vi "HydrophonePeaks.vi"() -> ()   [LabVIEW 2022 SP3]
uses:
  <vilib>/Analysis/NI_AALPro.lvlib
  <vilib>/Analysis/5stat.llb/RMS (DBL).vi
  <vilib>/Utility/file.llb/Write To Spreadsheet File (DBL).vi
panel:
  out "Waveform Graph 2":dbl[](graph)
  out "Waveform Graph":dbl[](graph)
  in  "file ext":string="*.eye"
  in  "Use Selected Files":bool
  in  "Listbox":i32[](listbox)
  in  "Choose Directory":path
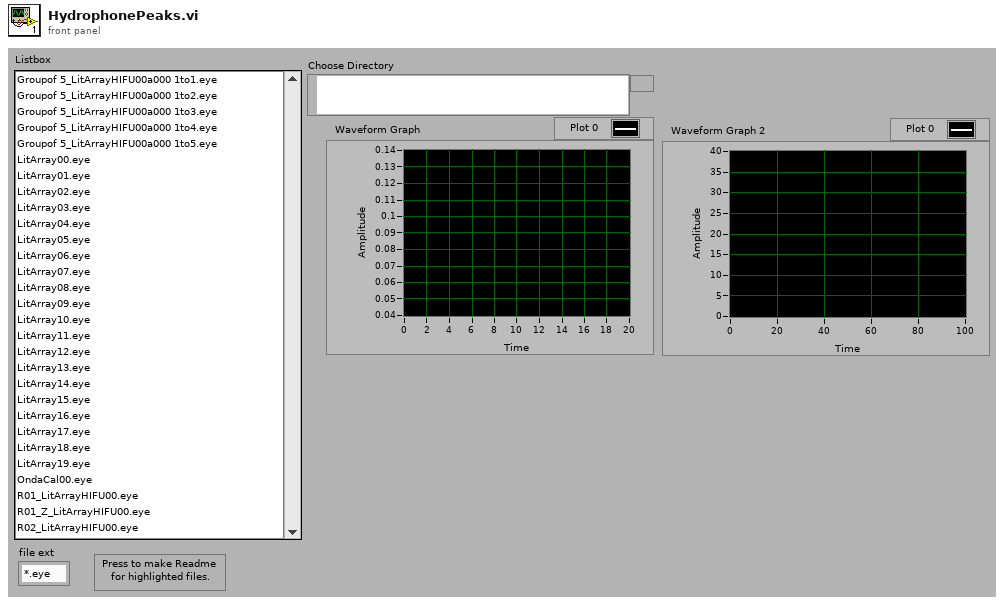
[diagram p1: front panel]
types:
  T1 = cluster{"Digitizer (dB)":sgl, "Gain (dB)":sgl, "Atten (dB)":sgl}
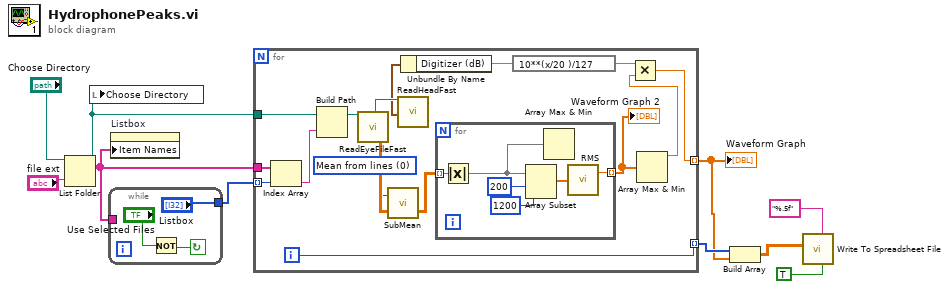
[diagram p0: block diagram]
diagram:
  n1 = List Folder(path="Choose Directory", pattern="file ext") -> (path out=w7:path, filenames=w10:string[])  [unwired: 1 in, 3 out]
  n2 = local write "Choose Directory"(w7) -> ()
  n3 = while {
    tunnel: ["Listbox"] -> w9
    tunnel: w10 -> [_]
    stop <- w13 continue-if-true
    n4 = Not(x="Use Selected Files") -> (.not. x?=w13:bool)
  }
  n5 = property on="Listbox" class="LstBox (strict)"("Item Names"=w10) -> ()  [unwired: 2 in, 2 out]
  n6 = for {
    tunnel: w10 -> [w29]
    tunnel: w9 -> [w28] mode=indexing
    tunnel: w7 -> [w26]
    tunnel: [w17] -> w4 mode=indexing
    tunnel: [w23] -> w5 mode=indexing
    i -> [w23]
    w14 = u16 0 items=["Mean from lines", "Mean just lines", "Poly Mean", "No mean"] ("Type of Mean")
    n7 = Index Array(array=w29, index=w28) -> (element=w27:string)
    n8 = Build Path(base path=w26, name or relative path=w27) -> (appended path=w25:path)
    n9 = call "ReadEyeFileFast.vi"("new file path"=w25) -> ("new path out"=w22:path, "2-D data array"=w15:sgl[][])  [unwired: 1 in, 16 out]
    n10 = call "SubMean.vi"("Scan Data In"=w15, "Type of Mean"=w14) -> ("Array"=w16:dbl[][])  [unwired: 1 out]
    n11 = call "ReadHeadFast.vi"("new file path"=w22) -> ("Votage scaling"=w21:T1)  [unwired: 2 in, 16 out]
    n12 = Unbundle By Name(w21) -> ("Digitizer (dB)"=w20:sgl)
    n13 = for {
      tunnel: w16 -> [w32] mode=indexing
      tunnel: [w30] -> w24 mode=indexing
      n14 = Absolute Value(x=w32) -> (abs(x)=w31:dbl[])
      n15 = Array Subset(array=w31, index=200, length=1200) -> (w33:dbl[])
      n16 = Array Max & Min(array=w31) -> ()  [unwired: 4 out]
      n17 = call-poly <vilib>:"RMS.vi"("X"=w33) -> ("rms value"=w30:dbl)  [unwired: 1 out]
    }
    "Waveform Graph 2" <- w24
    n18 = expression code="10**(x/20 )/127"(w20) -> (w19:sgl)
    n19 = Array Max & Min(array=w24) -> (max value=w18:dbl)  [unwired: 3 out]
    n20 = Multiply(x=w19, y=w18) -> (x*y=w17:dbl)
  }
  "Waveform Graph" <- w4
  n21 = Build Array(w5, w4) -> (w3:dbl[][])
  n22 = call-poly <vilib>:"Write To Spreadsheet File.vi"("transpose? (no:F)"=TRUE, "format (%.3f)"="%.5f", "2D data"=w3) -> ()  [unwired: 3 in, 3 out]
